vi "To and From CSV Test.vi"() -> (0 "error out":errorcluster, 1 "Pass":bool, 2 "Lines Equal":bool, 3 "Class Equal":bool)   [LabVIEW 2015, in "PID Module 2 tests.lvlib"]
uses:
  PID Module 2 tests.lvlib
  <vilib>/NI/Module Execution Interface/Engine Configuration/engine configuration.lvclass
  editor node/PID Module 2 editor node.lvclass
  module/configuration/PID Module 2 configuration.lvclass
  module/configuration/PID Module 2 configuration.lvclass/PID Module 2 configuration.ctl
  <vilib>/NI/Configuration Framework/serializable configuration/NISE_CEF_serializable configuration.lvclass/NISE_CEF_serializable configuration.ctl
  <vilib>/NI/Tag Bus/tag/tag descriptor.lvclass/tag descriptor.ctl
  <vilib>/NI/Tag Bus/tag/default value polymorphs/read default value Double.vi
  <vilib>/Utility/LVClass/Get LV Class Name.vi
  <vilib>/NI/Configuration Framework/error generator/NISE_error generator.vi
  <vilib>/NI/Tag Bus Module Framework/channel/TBM channel.lvclass
  <vilib>/NI/Configuration Framework/serializable configuration/NISE_CEF_serializable configuration.lvclass
  <vilib>/NI/Tag Bus/tag/tag descriptor.lvclass
panel:
  out "Array 8":string[](array[string])
  out "Array 7":string[](array[string])
  out "Array 6":string[](array[string])
  out "Array":string[](array[string])
  out "Array 5":string[][](array[string])
  out "Array 2":string[][](array[string])
  out "Array 4":string[](array[string])
  out "Array 3":string[](array[string])
  out "Write Channels":bool
  out "Read Channels":bool
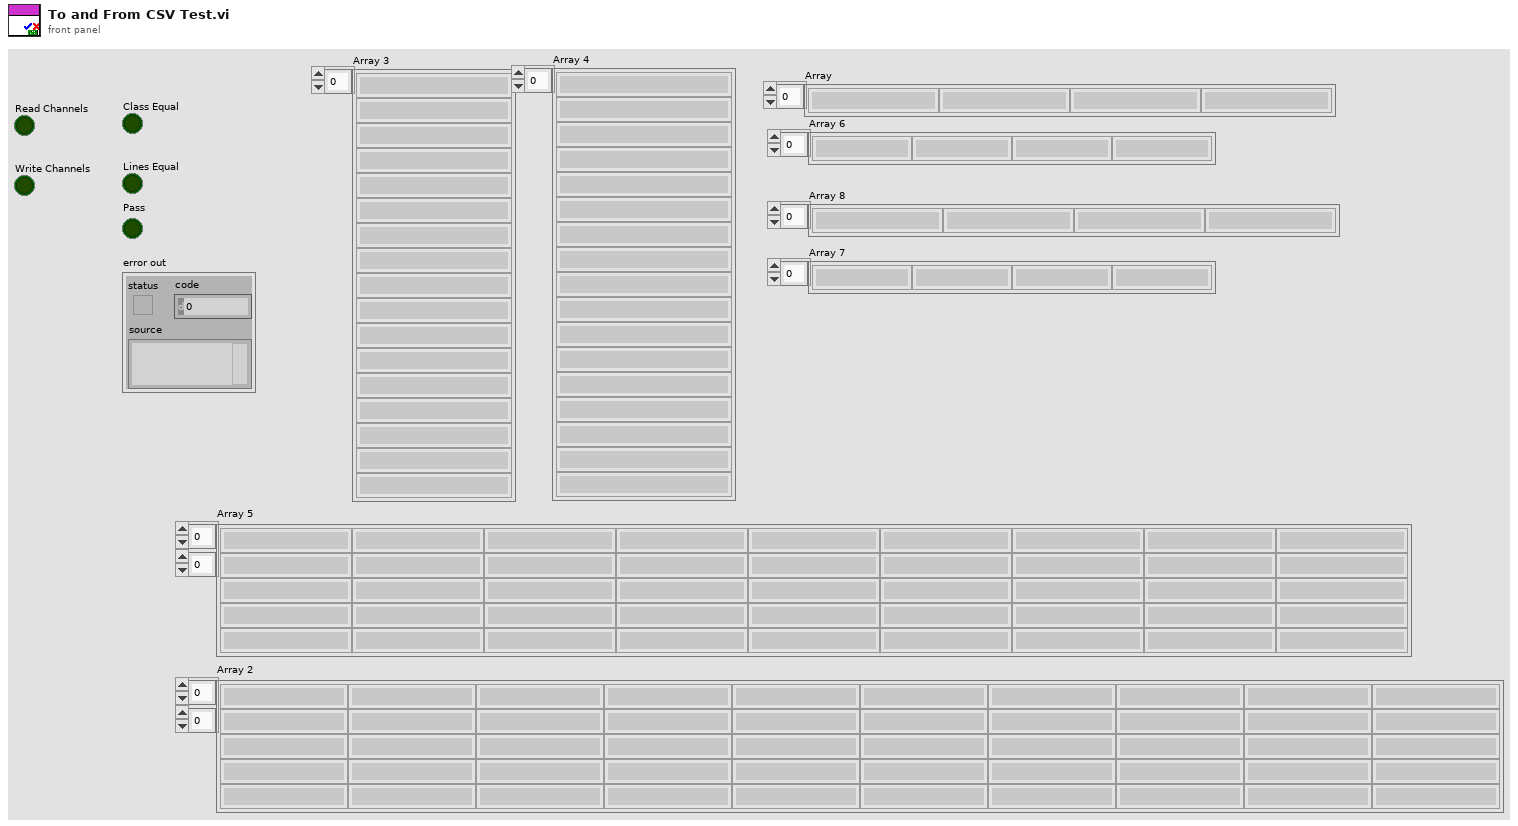
[diagram p1: front panel]
types:
  T1 = typedef "PID Module 2 configuration.lvclass/Line.ctl" = cluster{"PID ID":string, "Setpoint":refnum<class "TBM channel.lvclass">, "Variable":refnum<class "TBM channel.lvclass">, "Output":refnum<class "TBM channel.lvclass">, "Output High":refnum<class "TBM channel.lvclass">, "Output Low":refnum<class "TBM channel.lvclass">, "P":refnum<class "TBM channel.lvclass">, "I":refnum<class "TBM channel.lvclass">, "D":refnum<class "TBM channel.lvclass">}
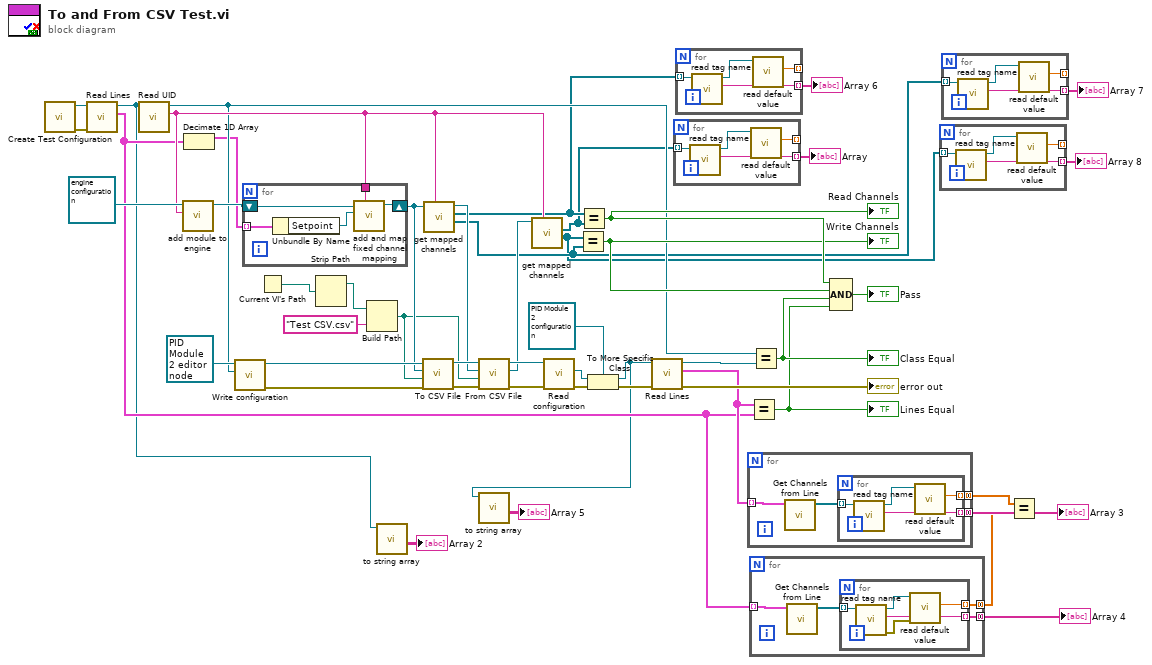
[diagram p0: block diagram]
diagram:
  n1 = call "Create Test Configuration.vi"() -> ("error out"=w49:errorcluster, "Module Configuration"=w50:refnum<class "PID Module 2 configuration.lvclass">)  [unwired: 6 in, 4 out]
  n2 = call "Read Lines.vi"("error in (no error)"=w49, "PID Module 2 configuration in"=w50) -> ("Lines"=w13:T1[], "PID Module 2 configuration out"=w11:refnum<class "PID Module 2 configuration.lvclass">)  [unwired: 7 in, 1 out]
  n3 = call <vilib>:"Read UID.vi"("configuration in"=w11) -> ("instance id"=w23:string, "configuration out"=w20:refnum<class "PID Module 2 configuration.lvclass">)  [unwired: 8 in, 1 out]
  n4 = call-dynamic "add module to engine.vi"("module ID"=w23, "engine configuration in"=refnum<class "engine configuration.lvclass"> refnum ("engine configuration")) -> ("engine configuration out"=w42:refnum<class "engine configuration.lvclass">)  [unwired: 8 in, 1 out]
  n5 = Decimate 1D Array(w13) -> (w19:T1[])  [unwired: 1 out]
  n6 = call-dynamic "Write configuration.vi"("configuration"=w20, "PID Module 2 editor node in"=refnum<class "PID Module 2 editor node.lvclass"> refnum ("tag bus configurable plugin editor node")) -> ("error out"=w36:errorcluster, "PID Module 2 editor node out"=w41:refnum<class "PID Module 2 editor node.lvclass">)  [unwired: 8 in]
  n7 = for {
    tunnel: w19 -> [w54] mode=indexing
    tunnel: w23 -> [w53]
    shift-right: [w52] -> w34
    shift-left: w42 -> [w51]
    n8 = Unbundle By Name(w54) -> ("Setpoint"=w55:refnum<class "TBM channel.lvclass">)
    n9 = call <vilib>:"add and map fixed channel mapping.vi"("module instance"=w53, "fixed channel"=w55, "engine configuration in"=w51) -> ("engine configuration out"=w52:refnum<class "engine configuration.lvclass">)  [unwired: 7 in, 1 out]
  }
  n10 = Current VI's Path() -> (path=w31:path)
  n11 = Strip Path(path=w31) -> (stripped path=w30:path)  [unwired: 1 out]
  n12 = Build Path(base path=w30, name or relative path="Test CSV.csv") -> (appended path=w29:path)
  n13 = call-dynamic "to string array.vi"("PID Module 2 configuration in"=w11) -> ("Array"=→"Array 2":string[][])  [unwired: 7 in, 3 out]
  n14 = call-dynamic "To CSV File.vi"("error in (no error)"=w36, "Path"=w29, "engine configuration"=w34, "PID Module 2 editor node in"=w41) -> ("error out"=w37:errorcluster, "PID Module 2 editor node out"=w39:refnum<class "PID Module 2 editor node.lvclass">)  [unwired: 6 in]
  n15 = call-dynamic "get mapped channels.vi"("owner"=w23, "engine configuration in"=w34) -> ("write channels"=w2:refnum<class "TBM channel.lvclass">[], "read channels"=w8:refnum<class "TBM channel.lvclass">[], "engine configuration out"=w33:refnum<class "engine configuration.lvclass">)  [unwired: 5 in, 2 out]
  n16 = call-dynamic "From CSV File.vi"("error in (no error)"=w37, "Path"=w29, "engine in"=w33, "PID Module 2 editor node in"=w39) -> ("error out"=w38:errorcluster, "engine out"=w28:refnum<class "engine configuration.lvclass">, "PID Module 2 editor node out"=w40:refnum<class "PID Module 2 editor node.lvclass">)  [unwired: 4 in, 1 out]
  n17 = call-dynamic "get mapped channels.vi"("owner"=w23, "engine configuration in"=w28) -> ("write channels"=w1:refnum<class "TBM channel.lvclass">[], "read channels"=w7:refnum<class "TBM channel.lvclass">[])  [unwired: 5 in, 3 out]
  n18 = call-dynamic "Read configuration.vi"("error in"=w38, "PID Module 2 editor node in"=w40) -> ("error out"=w25:errorcluster, "configuration"=w26:refnum<class "NISE_CEF_serializable configuration.lvclass">)  [unwired: 7 in, 1 out]
  n19 = Equal?(x=w1, y=w2) -> (x = y?=w43:bool)
  "Write Channels" <- w43
  n20 = Equal?(x=w8, y=w7) -> (x = y?=w44:bool)
  "Read Channels" <- w44
  n21 = To More Specific Class(target class=refnum<class "PID Module 2 configuration.lvclass"> refnum ("tag bus configurable plugin module configuration"), reference=w26, error in=w25) -> (specific class reference=w9:refnum<class "PID Module 2 configuration.lvclass">, error out=w24:errorcluster)
  n22 = call-dynamic "to string array.vi"("PID Module 2 configuration in"=w9) -> ("Array"=→"Array 5":string[][])  [unwired: 7 in, 3 out]
  n23 = call "Read Lines.vi"("error in (no error)"=w24, "PID Module 2 configuration in"=w9) -> ("error out"=→"error out":errorcluster, "Lines"=w14:T1[], "PID Module 2 configuration out"=w48:refnum<class "PID Module 2 configuration.lvclass">)  [unwired: 7 in]
  n24 = for {
    tunnel: w7 -> [w59] mode=indexing
    tunnel: [w58] -> w6 mode=indexing
    tunnel: [w56] -> _ mode=indexing
    n25 = call <vilib>:"read tag name.vi"("system tag in"=w59) -> ("name"=w58:string, "system tag out"=w57:refnum<class "TBM channel.lvclass">)  [unwired: 8 in, 1 out]
    n26 = call-poly <vilib>:"read default value.vi"("system tag in"=w57) -> ("default value"=w56:dbl)  [unwired: 7 in, 3 out]
  }
  "Array" <- w6
  n27 = for {
    tunnel: w8 -> [w63] mode=indexing
    tunnel: [w62] -> w5 mode=indexing
    tunnel: [w60] -> _ mode=indexing
    n28 = call <vilib>:"read tag name.vi"("system tag in"=w63) -> ("name"=w62:string, "system tag out"=w61:refnum<class "TBM channel.lvclass">)  [unwired: 8 in, 1 out]
    n29 = call-poly <vilib>:"read default value.vi"("system tag in"=w61) -> ("default value"=w60:dbl)  [unwired: 7 in, 3 out]
  }
  "Array 6" <- w5
  n30 = for {
    tunnel: w14 -> [w67] mode=indexing
    tunnel: [w65] -> w18 mode=concatenating
    tunnel: [w64] -> w16 mode=concatenating
    n31 = call "Get Channels from Line.vi"("Line"=w67) -> ("Channels"=w66:refnum<class "TBM channel.lvclass">[])  [unwired: 10 in]
    n32 = for {
      tunnel: w66 -> [w71] mode=indexing
      tunnel: [w70] -> w65 mode=indexing
      tunnel: [w68] -> w64 mode=indexing
      n33 = call <vilib>:"read tag name.vi"("system tag in"=w71) -> ("name"=w70:string, "system tag out"=w69:refnum<class "TBM channel.lvclass">)  [unwired: 8 in, 1 out]
      n34 = call-poly <vilib>:"read default value.vi"("system tag in"=w69) -> ("default value"=w68:dbl)  [unwired: 7 in, 3 out]
    }
  }
  "Array 3" <- w18
  n35 = Equal?(x=w14, y=w13) -> (x = y?=w21:bool)
  "Lines Equal" <- w21
  n36 = for {
    tunnel: w13 -> [w75] mode=indexing
    tunnel: [w73] -> w17 mode=concatenating
    tunnel: [w72] -> w15 mode=concatenating
    n37 = call "Get Channels from Line.vi"("Line"=w75) -> ("Channels"=w74:refnum<class "TBM channel.lvclass">[])  [unwired: 10 in]
    n38 = for {
      tunnel: w74 -> [w80] mode=indexing
      tunnel: [w79] -> w73 mode=indexing
      tunnel: [w76] -> w72 mode=indexing
      n39 = call <vilib>:"read tag name.vi"("system tag in"=w80) -> ("error out"=w78:errorcluster, "name"=w79:string, "system tag out"=w77:refnum<class "TBM channel.lvclass">)  [unwired: 8 in]
      n40 = call-poly <vilib>:"read default value.vi"("error in"=w78, "system tag in"=w77) -> ("default value"=w76:dbl)  [unwired: 6 in, 3 out]
    }
  }
  "Array 4" <- w17
  n41 = Equal?(x=w20, y=w48) -> (x = y?=w22:bool)
  "Class Equal" <- w22
  n42 = Compound Arithmetic op=AND(w44, w43, w22, w21) -> (→"Pass":bool)
  n43 = for {
    tunnel: w1 -> [w84] mode=indexing
    tunnel: [w83] -> w3 mode=indexing
    tunnel: [w81] -> _ mode=indexing
    n44 = call <vilib>:"read tag name.vi"("system tag in"=w84) -> ("name"=w83:string, "system tag out"=w82:refnum<class "TBM channel.lvclass">)  [unwired: 8 in, 1 out]
    n45 = call-poly <vilib>:"read default value.vi"("system tag in"=w82) -> ("default value"=w81:dbl)  [unwired: 7 in, 3 out]
  }
  "Array 8" <- w3
  n46 = for {
    tunnel: w2 -> [w88] mode=indexing
    tunnel: [w87] -> w4 mode=indexing
    tunnel: [w85] -> _ mode=indexing
    n47 = call <vilib>:"read tag name.vi"("system tag in"=w88) -> ("name"=w87:string, "system tag out"=w86:refnum<class "TBM channel.lvclass">)  [unwired: 8 in, 1 out]
    n48 = call-poly <vilib>:"read default value.vi"("system tag in"=w86) -> ("default value"=w85:dbl)  [unwired: 7 in, 3 out]
  }
  "Array 7" <- w4
  n49 = Equal?(x=w16, y=w15) -> ()  [unwired: 1 out]
